vi "xijk_automatic_read_folder.vi"(8 "error in":errorcluster, 11 "path in":path) -> (0 "error out":errorcluster, 2 "Filenames folders":path[](array[path]), 3 "Output filenames":path[](array[path]))   [LabVIEW 2010, in "xijk_automatic_read_and_guess.lvlib"]
uses:
  xijk_automatic_read_and_guess.lvlib
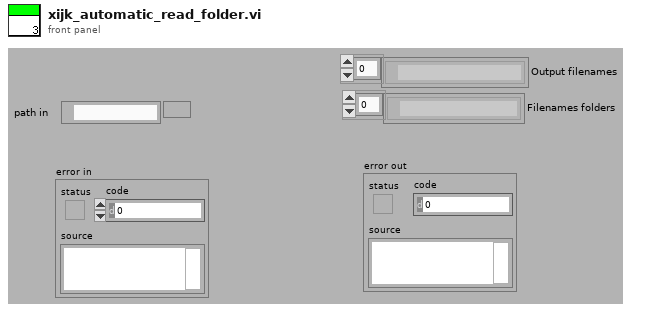
[diagram p1: front panel]
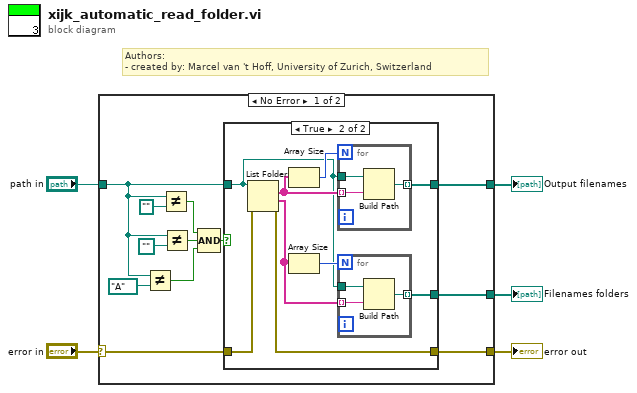
[diagram p0: block diagram]
diagram:
  # "Authors: \n- created by: Marcel van 't Hoff, University of Zurich, Switzerland"
  n1 = case shown="No Error" "error in" {
    selector: "error in" -> [w7 w34]
    tunnel: "path in" -> [w14 _]
    tunnel: [w9 _] -> w4
    tunnel: [w8 _] -> w3
    tunnel: [w6 w34] -> w1
    frame No Error {
      n2 = Not Equal?(x=w14, y=path "A:/" ("Chemin 2")) -> (x != y?=w11:bool)
      n3 = Not Equal?(x=w14, y=path "") -> (x != y?=w13:bool)
      n4 = Not Equal?(x=w14, y=path "") -> (x != y?=w12:bool)
      n5 = Compound Arithmetic op=AND(w13, w12, w11) -> (w10:bool)
      n6 = case shown="True" w10 {
        tunnel: w14 -> [_ w23]
        tunnel: [_ w22] -> w9
        tunnel: [_ w21] -> w8
        tunnel: w7 -> [w18 w20]
        tunnel: [w18 w19] -> w6
        frame False {
        }
        frame True {
          n7 = List Folder(path=w23, error in=w20) -> (filenames=w26:string[], folder names=w24:string[], error out=w19:errorcluster)  [unwired: 3 out]
          n8 = Array Size(array=w26) -> (size(s)=w27:i32)
          n9 = Array Size(array=w24) -> (size(s)=w25:i32)
          n10 = for {
            N: w27 -> [_]
            tunnel: w23 -> [w33]
            tunnel: w26 -> [w32] mode=indexing
            tunnel: [w31] -> w21 mode=indexing
            n11 = Build Path(base path=w33, name or relative path=w32) -> (appended path=w31:path)
          }
          n12 = for {
            N: w25 -> [_]
            tunnel: w23 -> [w30]
            tunnel: w24 -> [w29] mode=indexing
            tunnel: [w28] -> w22 mode=indexing
            n13 = Build Path(base path=w30, name or relative path=w29) -> (appended path=w28:path)
          }
        }
      }
    }
    frame Error {
    }
  }
  "Output filenames" <- w3
  "Filenames folders" <- w4
  "error out" <- w1
